vi "Lvdt Data Read.vi"() -> (1 "ng":bool, 2 "ok":bool)   [LabVIEW 2015]
uses:
  Galobal variable_TI.vi
  Project Setup/Globle Variable/GR_Servo.vi
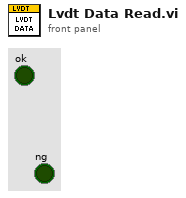
[diagram p1: front panel]
types:
  T1 = cluster{"Load Max(N)":dbl, "Load Min(N)":dbl, "Actuator1 max(mm)":dbl, "Actuator1min(mm)":dbl, "Actuator2 max(mm)":dbl, "Actuator2min(mm)":dbl, "Load Offset":dbl, "Model":string, "MIC Code":string}
  T2 = cluster{"Actuator1(mm)":dbl, "Actuator2(mm)":dbl, "Load(N)":dbl, "Actuator1":bool, "Actuator2":bool, "Load":bool}
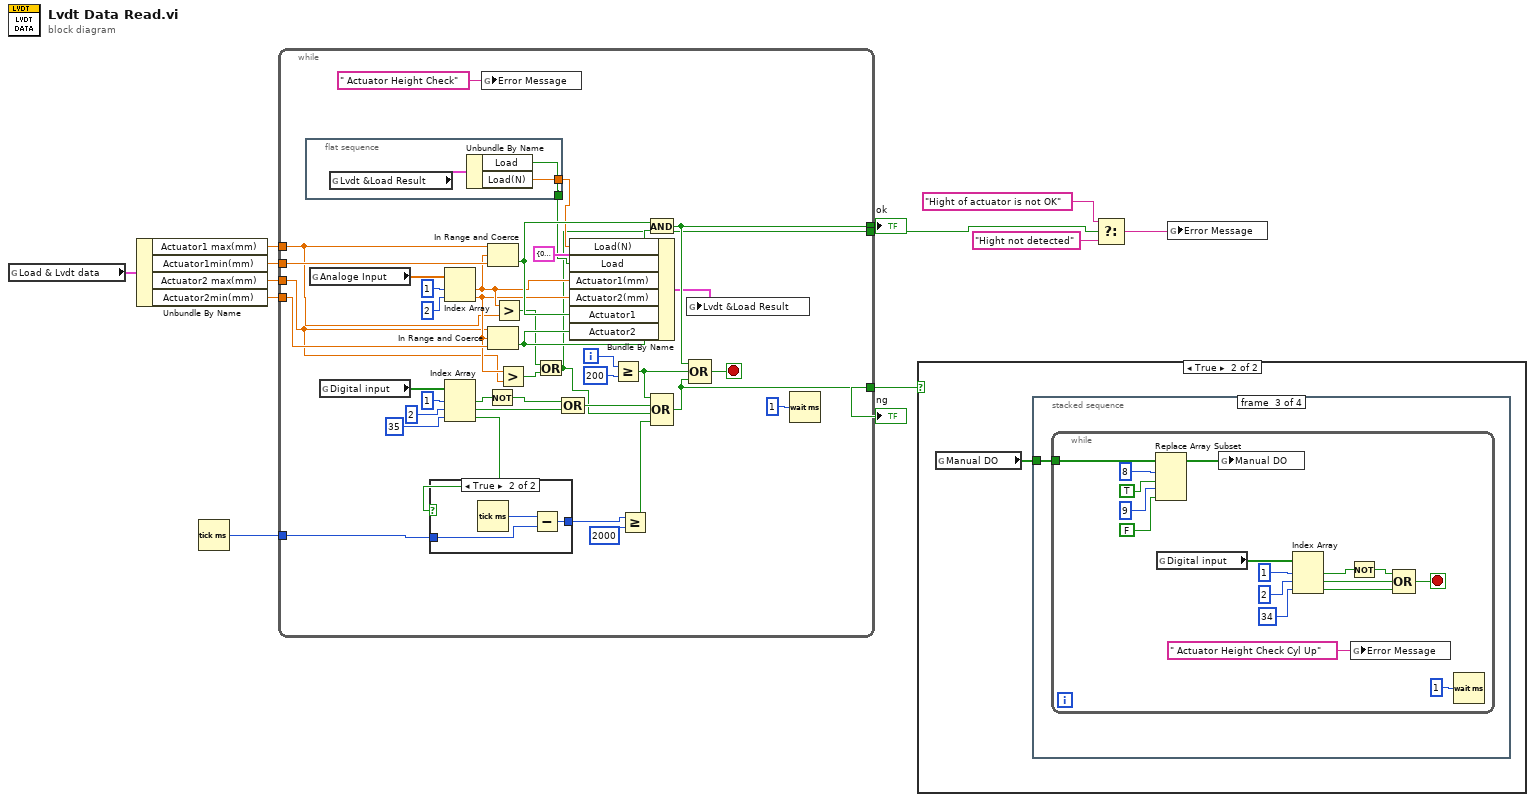
[diagram p0: block diagram]
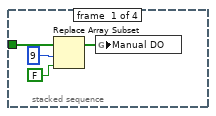
[diagram p3: hidden frame]
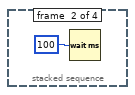
[diagram p4: hidden frame]
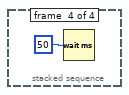
[diagram p5: hidden frame]
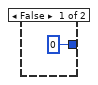
[diagram p6: hidden frame]
diagram:
  n1 = global read "Galobal variable_TI.vi" "Load & Lvdt data"() -> (w12:T1)
  n2 = Unbundle By Name(w12) -> ("Actuator1 max(mm)"=w11:dbl, "Actuator1min(mm)"=w10:dbl, "Actuator2 max(mm)"=w9:dbl, "Actuator2min(mm)"=w8:dbl)
  n3 = Tick Count (ms)() -> (millisecond timer value=w5:u32)
  n4 = while {
    tunnel: w11 -> [w26]
    tunnel: w10 -> [w45]
    tunnel: w9 -> [w25]
    tunnel: w8 -> [w44]
    tunnel: [w36] -> w7
    tunnel: [w34] -> w6
    tunnel: w5 -> [w20]
    tunnel: [w13] -> w4
    i -> [w50]
    stop <- w35 stop-if-true
    n5 = flat-sequence {
      tunnel: [w53] -> w15
      tunnel: [w52] -> w14
      frame #0 {
        n6 = global read "Galobal variable_TI.vi" "Lvdt &Load Result"() -> (w54:T2)
        n7 = Unbundle By Name(w54) -> ("Load"=w53:bool, "Load(N)"=w52:dbl)
      }
    }
    n8 = global read "Galobal variable_TI.vi" "Analoge Input"() -> (w48:dbl[])
    n9 = global read "Galobal variable_TI.vi" "Digital input"() -> (w38:bool[])
    n10 = Index Array(array=w48, index #1=1 ("index"), index #2=2 ("index")) -> (element #1=w28:dbl, element #2=w27:dbl)
    n11 = Index Array(array=w38, index #1=1 ("index"), index #2=2 ("index"), index #3=35 ("index")) -> (element #1=w41:bool, element #2=w39:bool, element #3=w17:bool)
    n12 = case shown="True" w17 {
      tunnel: w20 -> [_ w57]
      tunnel: [u32 0 w56] -> w22
      frame False {
      }
      frame True {
        n13 = Tick Count (ms)() -> (millisecond timer value=w58:u32)
        n14 = Subtract(x=w58, y=w57) -> (x-y=w56:u32)
      }
    }
    n15 = global write "GR_Servo.vi" "Error Message"(" Actuator Height Check") -> ()
    n16 = Not(x=w41) -> (.not. x?=w40:bool)
    n17 = In Range and Coerce(upper limit=w26, x=w28, lower limit=w45) -> (In Range?=w32:bool)  [unwired: 1 out]
    n18 = In Range and Coerce(upper limit=w25, x=w27, lower limit=w44) -> (In Range?=w31:bool)  [unwired: 1 out]
    n19 = Greater?(x=w28, y=w26) -> (0:w24:bool)
    n20 = Greater?(x=w27, y=w25) -> (0:w23:bool)
    n21 = Or(x=w24, y=w23) -> (x .or. y?=w13:bool)
    n22 = Compound Arithmetic op=OR(w40, w39) -> (w37:bool)
    n23 = Bundle By Name(cluster=T2 {"Actuator1(mm)"=0.0, "Actuator2(mm)"=0.0, "Load(N)"=0.0, "Actuator1"=FALSE, "Actuator2"=FALSE, "Load"=FALSE} ("Lvdt &Load Result"), "Load(N)"=w14, "Load"=w15, "Actuator1(mm)"=w28, "Actuator2(mm)"=w27, "Actuator1"=w32, "Actuator2"=w31) -> (w30:T2)
    n24 = Greater Or Equal?(x=w50, y=200) -> (x >= y?=w43:bool)
    n25 = Greater Or Equal?(x=w22, y=u32 2000) -> (x >= y?=w16:bool)
    n26 = And(x=w32, y=w31) -> (x .and. y?=w36:bool)
    n27 = Compound Arithmetic op=OR(w43, w37, w13, w16) -> (w34:bool)
    n28 = global write "Galobal variable_TI.vi" "Lvdt &Load Result"(w30) -> ()
    n29 = Compound Arithmetic op=OR(w36, w43, w34) -> (w35:bool)
    n30 = Wait (ms)(milliseconds to wait=u32 1) -> ()  [unwired: 1 out]
  }
  "ok" <- w7
  "ng" <- w6
  n31 = case shown="True" w6 {
    frame False {
    }
    frame True {
      n32 = global read "Galobal variable_TI.vi" "Manual DO"() -> (w59:bool[])
      n33 = stacked-sequence {
        tunnel: w59 -> [w63 _ w65 _]
        frame #0 {
          n34 = Replace Array Subset(array=w63, new element=FALSE ("new element/subarray"), index=9) -> (w60:bool[])
          n35 = global write "Galobal variable_TI.vi" "Manual DO"(w60) -> ()
        }
        frame #1 {
          n36 = Wait (ms)(milliseconds to wait=u32 100) -> ()  [unwired: 1 out]
        }
        frame #2 {
          n37 = while {
            tunnel: w65 -> [w80]
            stop <- w68 stop-if-true
            n38 = Replace Array Subset(array=w80, new element #1=TRUE ("new element/subarray"), index #1=8 ("index"), new element #2=FALSE ("new element/subarray"), index #2=9 ("index")) -> (w79:bool[])
            n39 = global read "Galobal variable_TI.vi" "Digital input"() -> (w73:bool[])
            n40 = global write "Galobal variable_TI.vi" "Manual DO"(w79) -> ()
            n41 = Index Array(array=w73, index #1=1 ("index"), index #2=2 ("index"), index #3=34 ("index")) -> (element #1=w77:bool, element #2=w74:bool, element #3=w71:bool)
            n42 = Not(x=w77) -> (.not. x?=w75:bool)
            n43 = global write "GR_Servo.vi" "Error Message"(" Actuator Height Check Cyl Up") -> ()
            n44 = Compound Arithmetic op=OR(w75, w74, w71) -> (w68:bool)
            n45 = Wait (ms)(milliseconds to wait=u32 1) -> ()  [unwired: 1 out]
          }
        }
        frame #3 {
          n46 = Wait (ms)(milliseconds to wait=u32 50) -> ()  [unwired: 1 out]
        }
      }
    }
  }
  n47 = Select(t="Hight of actuator is not OK", s=w4, f="Hight not detected") -> (s? t:f=w2:string)
  n48 = global write "GR_Servo.vi" "Error Message"(w2) -> ()
